vi "go_to_user_defined_temp.vi"(0 "VISA resource name":refnum<visa-resource-name>, 2 "Status  Control":bool, 11 "error in (no error)":errorcluster, 13 "Target Temperature / K":dbl=4.5 min=4.5 max=500.0 step=1.0) -> (4 "VISA resource name out":refnum<visa-resource-name>, 15 "error out":errorcluster)   [LabVIEW 2023]
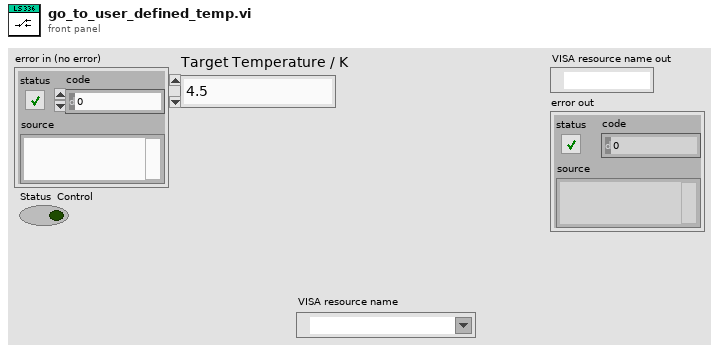
[diagram p1: front panel]
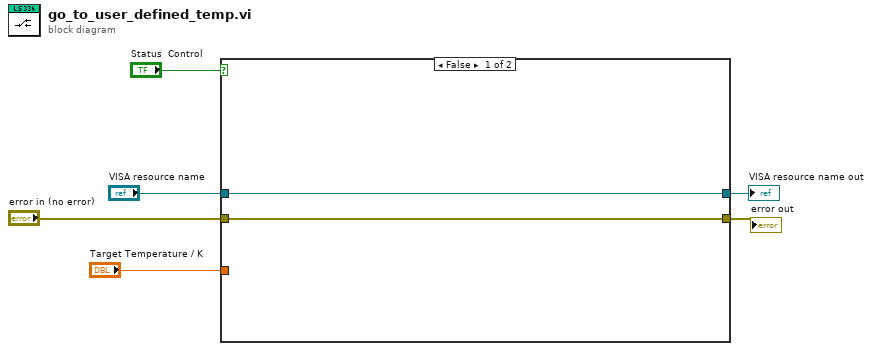
[diagram p0: block diagram]
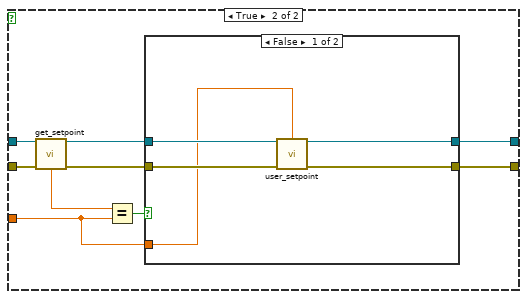
[diagram p2: hidden frame]
diagram:
  n1 = case shown="False" "Status  Control" {
    tunnel: "VISA resource name" -> [w8 w17]
    tunnel: "error in (no error)" -> [w7 w16]
    tunnel: "Target Temperature / K" -> [_ w11]
    tunnel: [w8 w10] -> w3
    tunnel: [w7 w9] -> w2
    frame False {
    }
    frame True {
      n2 = call "get_setpoint.vi"("VISA resource name"=w17, "error in (no error)"=w16) -> ("VISA resource name out"=w15:refnum<visa-resource-name>, "Current Setpoint / K"=w13:dbl, "error out"=w14:errorcluster)  [unwired: 11 in]
      n3 = Equal?(x=w13, y=w11) -> (x = y?=w12:bool)
      n4 = case shown="False" w12 {
        tunnel: w15 -> [w22 w24]
        tunnel: w14 -> [w19 w23]
        tunnel: [w20 w24] -> w10
        tunnel: [w21 w23] -> w9
        tunnel: w11 -> [w18 _]
        frame False {
          n5 = call "user_setpoint.vi"("VISA resource name"=w22, "Setpoint / K"=w18, "error in (no error)"=w19) -> ("VISA resource name out"=w20:refnum<visa-resource-name>, "error out"=w21:errorcluster)  [unwired: 11 in]
        }
        frame True {
        }
      }
    }
  }
  "VISA resource name out" <- w3
  "error out" <- w2
